vi "DatosAcelerometroHTCM9.vi"() -> ()   [LabVIEW 2018]
uses:
  <vilib>/Instr/_visa.llb/VISA Configure Serial Port (Instr).vi
panel:
  out "Z Axis Cambio":dbl
  out "Y Axis Cambio":dbl
  out "X Axis Cambio":dbl
  out "Waveform Chart Acelerometro":cluster{i32, i32, i32}(graph)
  out "String":string
  out "Z Axis":dbl
  out "Y Axis":dbl
  out "X Axis":dbl
  in  "stop":bool
  out "read buffer":string
  in  "baud rate (9600)":u32=9600
  in  "VISA resource name":refnum<visa-resource-name>
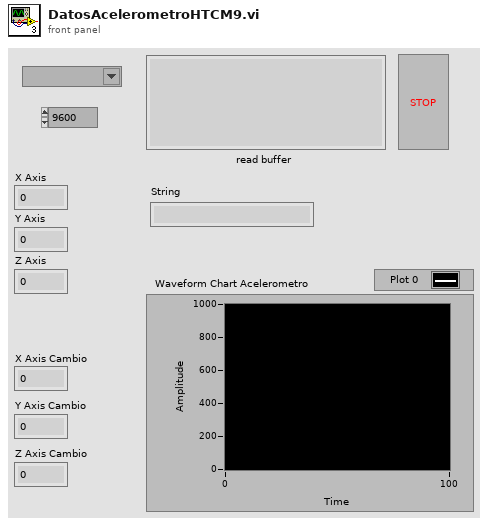
[diagram p1: front panel]
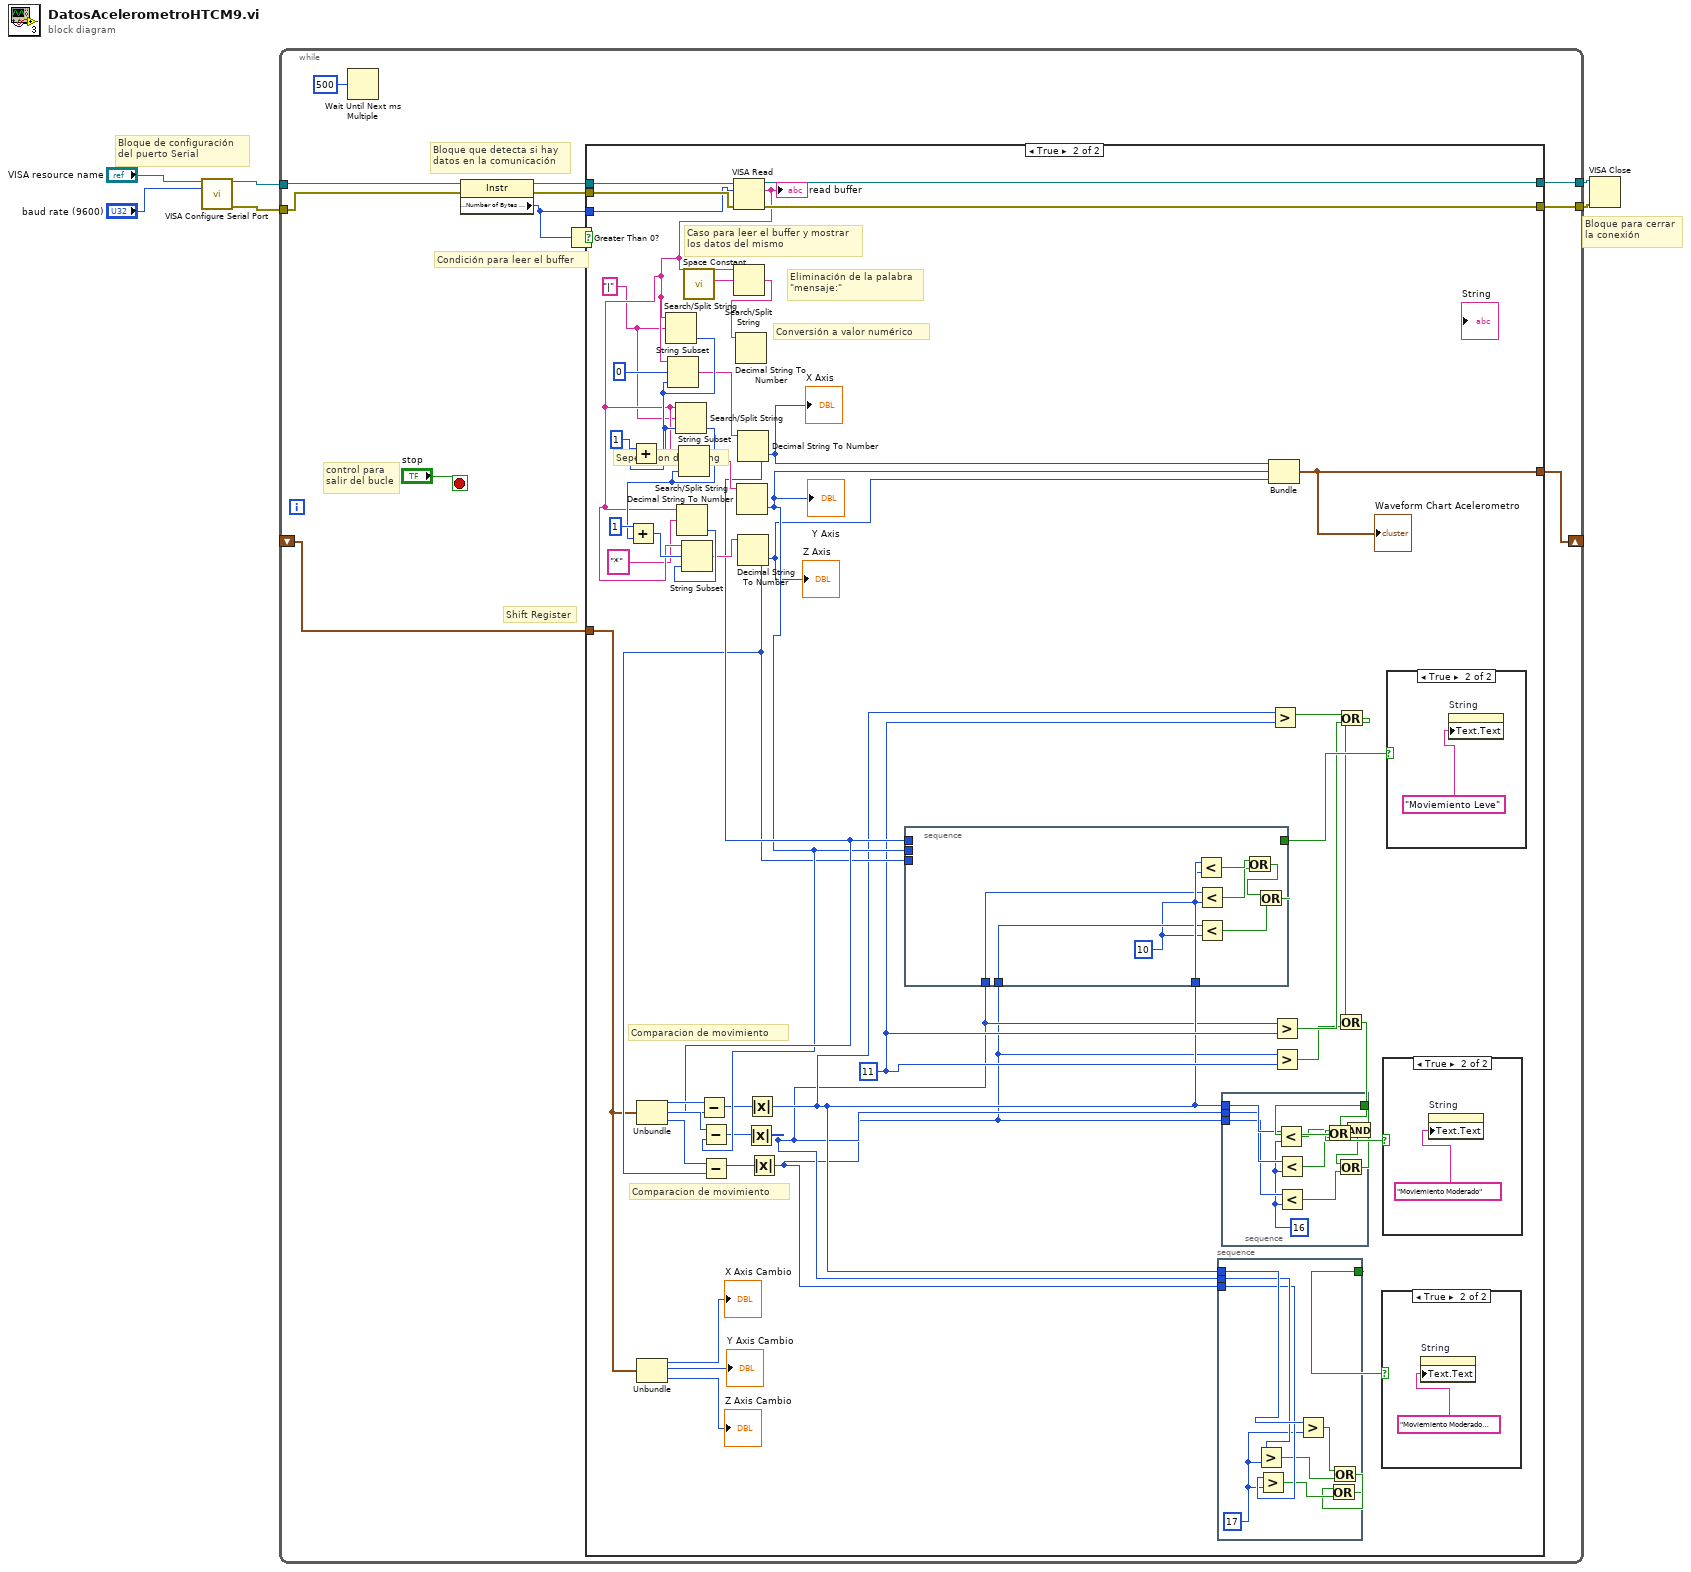
[diagram p0: block diagram]
diagram:
  # "Bloque de configuración\ndel puerto Serial"
  # "Bloque para cerrar\nla conexión"
  n1 = call-poly "VISA Configure Serial Port"("VISA resource name"="VISA resource name", "baud rate (9600)"="baud rate (9600)") -> ("VISA resource name out"=w1:refnum<visa-resource-name>, "error out"=w2:errorcluster)  [unwired: 12 in]
  n2 = while {
    tunnel: w1 -> [w9]
    tunnel: w2 -> [w10]
    tunnel: [w15] -> w4
    tunnel: [w14] -> w3
    shift-right: [w8] -> _
    shift-left: _ -> [w7]
    stop <- "stop" stop-if-true
    # "Shift Register"
    # "control para\nsalir del bucle"
    # "Bloque que detecta si hay\ndatos en la comunicación"
    # "Condición para leer el buffer"
    n3 = Wait Until Next ms Multiple(millisecond multiple=u32 500) -> ()  [unwired: 1 out]
    n4 = property class="Instr"(reference=w9, error in=w10) -> (reference out=w16:refnum<visa-resource-name>, error out=w17:errorcluster, "Serial Settings:Number of Bytes at Serial Port"=w11:u32)
    n5 = Greater Than 0?(x=w11) -> (x > 0?=w18:bool)
    n6 = case shown="True" w18 {
      tunnel: w17 -> [w19 w68]
      tunnel: w16 -> [w20 w67]
      tunnel: [w19 w66] -> w15
      tunnel: [w20 w65] -> w14
      tunnel: w11 -> [_ w64]
      tunnel: [_ w38] -> w8
      tunnel: w7 -> [_ w33]
      frame False {
        # "Este es el caso donde no hay \ndatos en la comunicación"
      }
      frame True {
        w29 = 11
        w49 = "|"
        # "Comparacion de movimiento"
        # "Seperacion del String"
        # "Comparacion de movimiento"
        # "Conversión a valor numérico"
        # "Eliminación de la palabra\n\"mensaje:\""
        # "Caso para leer el buffer y mostrar\nlos datos del mismo"
        n7 = Unbundle(w33) -> (w46:i32, w45:i32, w44:i32)
        n8 = Unbundle(w33) -> (→"X Axis Cambio":i32, →"Y Axis Cambio":i32, →"Z Axis Cambio":i32)
        n9 = call <vilib>:"Space Constant.vi"() -> ("String"=w63:string)
        n10 = VISA Read(VISA resource name=w67, byte count=w64, error in (no error)=w68) -> (VISA resource name out=w65:refnum<visa-resource-name>, read buffer=w50:string, error out=w66:errorcluster)  [unwired: 1 out]
        "read buffer" <- w50
        n11 = Search/Split String(string=w50, search string/char (-)=w49) -> (offset of match=w59:i32)  [unwired: 1 in, 2 out]
        n12 = Add(x=1, y=w59) -> (x+y=w58:i32)
        n13 = String Subset(string=w50, offset (0)=0, length (rest)=w59) -> (substring=w53:string)
        n14 = Search/Split String(string=w50, search string/char (-)=w49, offset (0)=w58) -> (offset of match=w56:i32)  [unwired: 2 out]
        n15 = Add(x=1, y=w56) -> (x+y=w55:i32)
        n16 = Search/Split String(string=w50, search string/char (-)="*") -> (offset of match=w54:i32)  [unwired: 1 in, 2 out]
        n17 = String Subset(string=w50, offset (0)=w58, length (rest)=w56) -> (substring=w52:string)
        n18 = String Subset(string=w50, offset (0)=w55, length (rest)=w54) -> (substring=w51:string)
        n19 = Search/Split String(string=w50, search string/char (-)=w63) -> (match + rest of string=w62:string)  [unwired: 1 in, 2 out]
        n20 = Decimal String To Number(string=w62) -> ()  [unwired: 2 in, 2 out]
        n21 = Decimal String To Number(string=w52) -> (number=w41:i32)  [unwired: 2 in, 1 out]
        "Y Axis" <- w41
        n22 = Subtract(x=w45, y=w41) -> (x-y=w36:i32)
        n23 = Decimal String To Number(string=w53) -> (number=w42:i32)  [unwired: 2 in, 1 out]
        "X Axis" <- w42
        n24 = Subtract(x=w46, y=w42) -> (x-y=w37:i32)
        n25 = Decimal String To Number(string=w51) -> (number=w40:i32)  [unwired: 2 in, 1 out]
        "Z Axis" <- w40
        n26 = Subtract(x=w44, y=w40) -> (x-y=w35:i32)
        n27 = Absolute Value(x=w36) -> (abs(x)=w22:i32)
        n28 = Absolute Value(x=w37) -> (abs(x)=w23:i32)
        n29 = Absolute Value(x=w35) -> (abs(x)=w21:i32)
        n30 = stacked-sequence {
          tunnel: [w73] -> w47
          tunnel: w40 -> [_]
          tunnel: w41 -> [_]
          tunnel: w42 -> [_]
          tunnel: w23 -> [w72]
          tunnel: w22 -> [w71]
          tunnel: w21 -> [w70]
          frame #0 {
            w69 = 10
            n31 = Less?(x=w72, y=w69) -> (x < y?=w77:bool)
            n32 = Less?(x=w71, y=w69) -> (x < y?=w76:bool)
            n33 = Less?(x=w70, y=w69) -> (x < y?=w74:bool)
            n34 = Or(x=w77, y=w76) -> (x .or. y?=w75:bool)
            n35 = Or(x=w75, y=w74) -> (x .or. y?=w73:bool)
          }
        }
        n36 = stacked-sequence {
          tunnel: [w78] -> w34
          tunnel: w21 -> [w84]
          tunnel: w22 -> [w85]
          tunnel: w23 -> [w86]
          frame #0 {
            w83 = 17
            n37 = Greater?(x=w85, y=w83) -> (0:w81:bool)
            n38 = Greater?(x=w84, y=w83) -> (0:w80:bool)
            n39 = Greater?(x=w86, y=w83) -> (0:w82:bool)
            n40 = Or(x=w82, y=w81) -> (x .or. y?=w79:bool)
            n41 = Or(x=w79, y=w80) -> (x .or. y?=w78:bool)
          }
        }
        n42 = stacked-sequence {
          tunnel: [w87] -> w43
          tunnel: w21 -> [w93]
          tunnel: w22 -> [w94]
          tunnel: w23 -> [w95]
          frame #0 {
            w92 = 16
            n43 = Less?(x=w95, y=w92) -> (x < y?=w89:bool)
            n44 = Less?(x=w94, y=w92) -> (x < y?=w90:bool)
            n45 = Less?(x=w93, y=w92) -> (x < y?=w91:bool)
            n46 = Or(x=w89, y=w90) -> (x .or. y?=w88:bool)
            n47 = Or(x=w88, y=w91) -> (x .or. y?=w87:bool)
          }
        }
        n48 = Bundle(w42, w41, w40) -> (w38:cluster{i32, i32, i32})  [unwired: 1 in]
        "Waveform Chart Acelerometro" <- w38
        n49 = Greater?(x=w23, y=w29) -> (0:w27:bool)
        n50 = Greater?(x=w22, y=w29) -> (0:w28:bool)
        n51 = Greater?(x=w21, y=w29) -> (0:w26:bool)
        n52 = Or(x=w27, y=w28) -> (x .or. y?=w25:bool)
        n53 = Or(x=w25, y=w26) -> (x .or. y?=w24:bool)
        n54 = And(x=w24, y=w43) -> (x .and. y?=w39:bool)
        n55 = case shown="True" w34 {
          frame False {
          }
          frame True {
            n56 = property on="String" class="Str"("Text.Text"="Moviemiento Moderado Fuerte") -> ()  [unwired: 2 in, 2 out]
          }
        }
        n57 = case shown="True" w39 {
          frame False {
          }
          frame True {
            n58 = property on="String" class="Str"("Text.Text"="Moviemiento Moderado") -> ()  [unwired: 2 in, 2 out]
          }
        }
        n59 = case shown="True" w47 {
          frame False {
          }
          frame True {
            n60 = property on="String" class="Str"("Text.Text"="Moviemiento Leve") -> ()  [unwired: 2 in, 2 out]
          }
        }
      }
    }
  }
  n61 = VISA Close(VISA resource name=w3, error in (no error)=w4) -> ()  [unwired: 1 out]
